vi "Display results.vi"(0 "Cluster":cluster{"Spots":i32[], "Average time":dbl[]}) -> ()   [LabVIEW 8.6]
uses:
  <vilib>/Utility/file.llb/Write To Spreadsheet File (DBL).vi
panel:
  in  "Save data?":bool
  in  "stop":bool
  out "XY Graph":cluster{"Array 2":i32[], "Array 3":dbl[]}(graph)
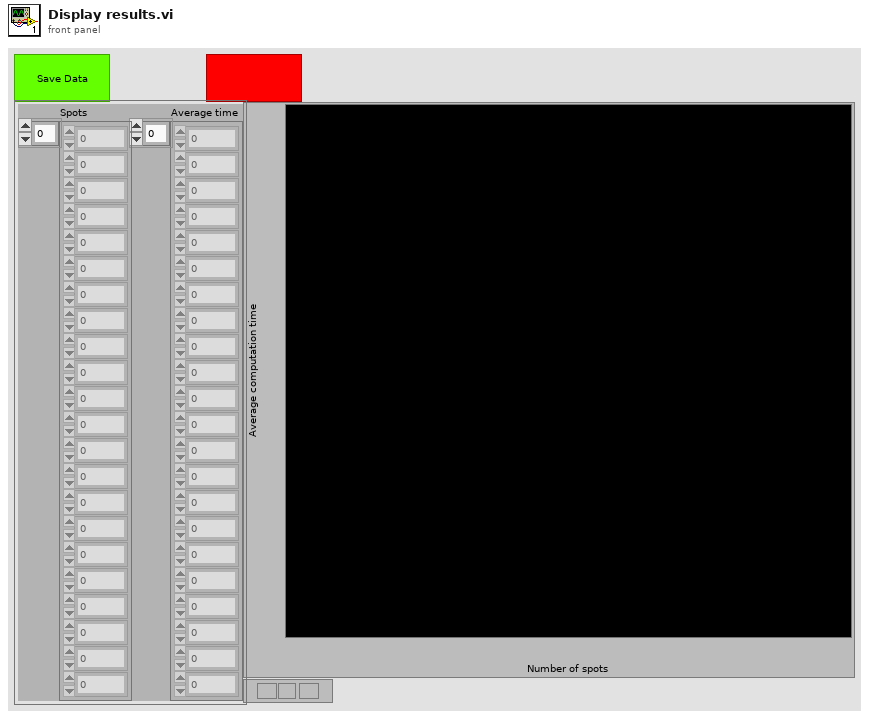
[diagram p1: front panel]
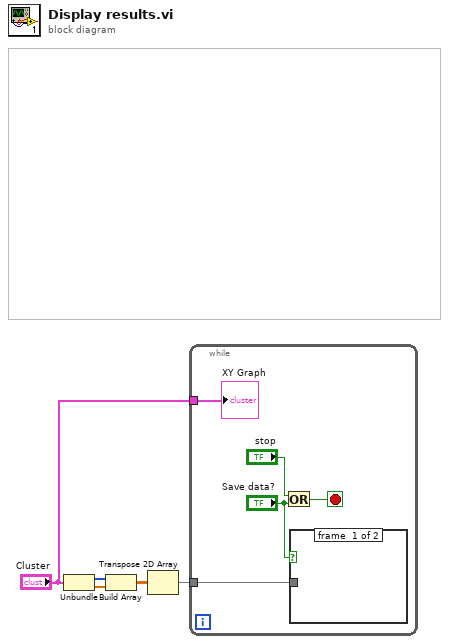
[diagram p0: block diagram]
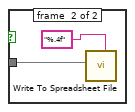
[diagram p2: hidden frame]
diagram:
  n1 = Unbundle("Cluster") -> ("Spots"=w2:i32[], "Average time"=w1:dbl[])
  n2 = Build Array(w2, w1) -> (w4:dbl[][])
  n3 = Transpose 2D Array(2D array=w4) -> (transposed array=w5:dbl[][])
  n4 = while {
    tunnel: w5 -> [w10]
    tunnel: "Cluster" -> [w8]
    stop <- w9 stop-if-true
    n5 = Or(x="stop", y="Save data?") -> (x .or. y?=w9:bool)
    n6 = case shown="True" "Save data?" {
      tunnel: w10 -> [_ w12]
      frame #0 {
      }
      frame #1 {
        n7 = call-poly <vilib>:"Write To Spreadsheet File.vi"("format (%.3f)"="%.4f", "2D data"=w12) -> ()  [unwired: 6 in, 1 out]
      }
    }
    "XY Graph" <- w8
  }
